vi "transition est.vi"(7 "bit":bool) -> (4 "p12":dbl, 6 "p21":dbl)   [LabVIEW 2017]
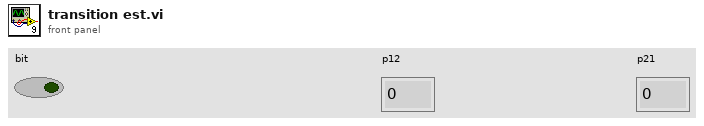
[diagram p1: front panel]
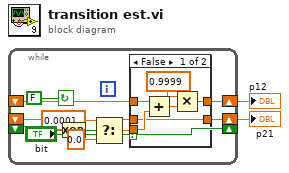
[diagram p0: block diagram]
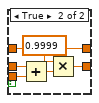
[diagram p2: hidden frame]
diagram:
  n1 = while {
    shift-right: ["bit"] -> _
    shift-left: _ -> [w11]
    shift-right: [w6] -> w1
    shift-left: _ -> [w5]
    shift-right: [w4] -> w2
    shift-left: _ -> [w3]
    stop <- FALSE continue-if-true
    n2 = Exclusive Or(1:"bit", 2:w11) -> (0:w10:bool)
    n3 = Select(t=0.0001, s=w10, f=0.0) -> (s? t:f=w7:dbl)
    n4 = case shown="False" "bit" {
      tunnel: w7 -> [w17 w25]
      tunnel: [w14 w24] -> w6
      tunnel: w5 -> [w14 w23]
      tunnel: [w19 w22] -> w4
      tunnel: w3 -> [w18 w22]
      frame False {
        n5 = Add(x=w18, y=w17) -> (x+y=w16:dbl)
        n6 = Multiply(x=0.9999 ("y"), y=w16) -> (x*y=w19:dbl)
      }
      frame True {
        n7 = Add(x=w23, y=w25) -> (x+y=w21:dbl)
        n8 = Multiply(x=0.9999 ("y"), y=w21) -> (x*y=w24:dbl)
      }
    }
  }
  "p12" <- w2
  "p21" <- w1
